vi "webpub.vi"() -> ()   [LabVIEW 2010]
uses:
  <vilib>/Analysis/NI_AALBase.lvlib
panel:
  in  "幅值":dbl(slide)=2.67175572519084 scale=0.0..10.0
  out "波形图":dbl[](graph)
  in  "停止":bool
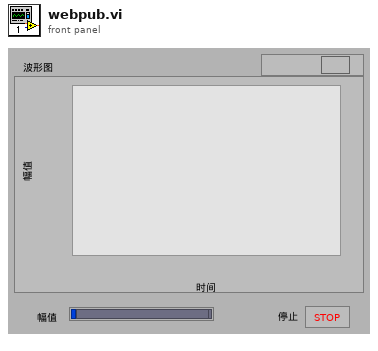
[diagram p1: front panel]
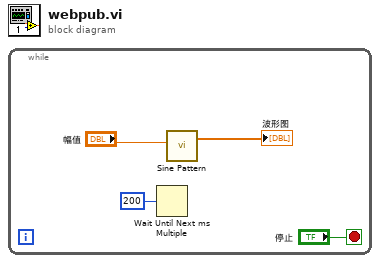
[diagram p0: block diagram]
diagram:
  n1 = while {
    stop <- "停止" stop-if-true
    n2 = Wait Until Next ms Multiple(millisecond multiple=u32 200) -> ()  [unwired: 1 out]
    n3 = call <vilib>:"Sine Pattern.vi"("amplitude"="幅值") -> ("Sinusoidal Pattern"=→"波形图":dbl[])  [unwired: 3 in, 1 out]
  }
